vi "KM_appendline.vi"(4 "Time (s)":dbl, 6 "name or relative path":string, 7 "read/write control":T3, 8 "Field":dbl, 9 "temperature":dbl, 10 "pm lorentzian":T1={"Amplitude"=nan, "omega(0)"=47559.741592685685, "Gamma"=1.85203362605106e-05, "phase"=nan, "Q"=2567973978.6417074, "Norm  Ampl"=nan, "z (inf)"=nan+nani, "4corners"={"z (-pi/2)"=nan+nani, "z(inf)"=nan+nani, "z (pi/2)"=nan+nani, "z center"=nan+nani, "z(0)"=nan+nani, "radius"=nan}} {"z (inf)" format="%#9_9f"; "Q" format="%#9_9f"; "phase" format="%#9_9f"; "Gamma" format="%#9_9f"; "omega(0)" format="%#9_9f"}, 11 "Save frequency scan":path=path "C:/data/Ultrasound/birdcage/Hg1201/Test") -> ()   [LabVIEW 2016]
uses:
  KM_file -- read-write control.ctl
  lorentzian.ctl
  circle corners.ctl
  file -- read-write control.ctl
  <vilib>/Utility/libraryn.llb/Check if File or Folder Exists.vi
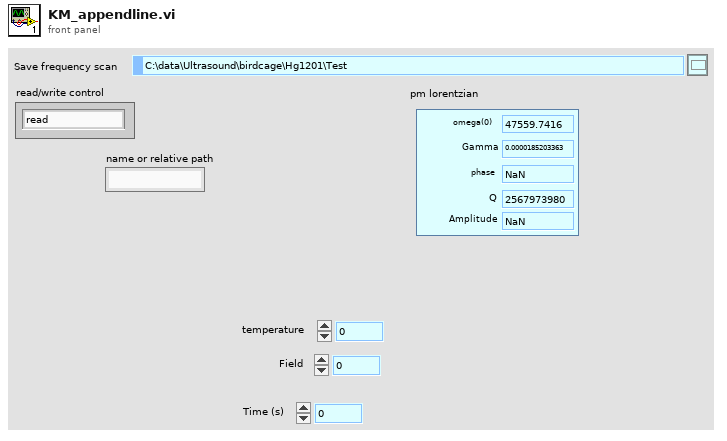
[diagram p1: front panel]
types:
  T1 = typedef "lorentzian.ctl" = cluster{"Amplitude":dbl, "omega(0)":dbl, "Gamma":dbl, "phase":dbl, "Q":dbl, "Norm  Ampl":dbl, "z (inf)":cdb, "4corners":T2}
  T2 = typedef "circle corners.ctl" = cluster{"z (-pi/2)":cdb, "z(inf)":cdb, "z (pi/2)":cdb, "z center":cdb, "z(0)":cdb, "radius":dbl}
  T3 = typedef "KM_file -- read-write control.ctl" = enum16{"read", "write all", "append one line"}
  T4 = typedef "file -- read-write control.ctl" = enum16{"read", "write all", "append one line"}
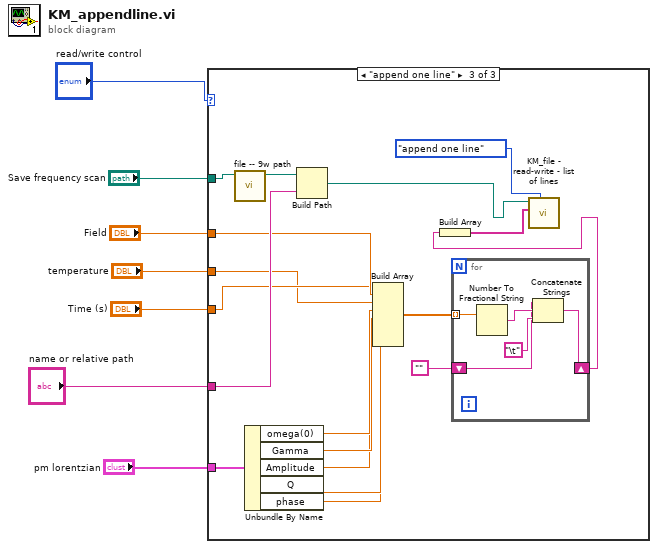
[diagram p0: block diagram]
diagram:
  n1 = case shown="\"append one line\"" "read/write control" {
    tunnel: "Save frequency scan" -> [_ _ w25]
    tunnel: "name or relative path" -> [_ _ w23]
    tunnel: "pm lorentzian" -> [_ _ w22]
    tunnel: "Field" -> [_ _ w21]
    tunnel: "Time (s)" -> [_ _ w20]
    tunnel: "temperature" -> [_ _ w19]
    frame "read", Default {
    }
    frame "write all" {
    }
    frame "append one line" {
      n2 = call "file -- 9w path.vi"("sweep folder"=w25) -> ("9w path"=w24:path)  [unwired: 10 in]
      n3 = Unbundle By Name(w22) -> ("omega(0)"=w18:dbl, "Gamma"=w17:dbl, "Amplitude"=w16:dbl, "Q"=w15:dbl, "phase"=w14:dbl)
      n4 = Build Path(base path=w24, name or relative path=w23) -> (appended path=w9:path)
      n5 = Build Array(w20, w21, w19, w18, w17, w16, w15, w14) -> (w13:dbl[])
      n6 = for {
        tunnel: w13 -> [w30] mode=indexing
        shift-right: [w26] -> w11
        shift-left: "" -> [w27]
        n7 = Number To Fractional String(number=w30) -> (F-format string=w29:string)  [unwired: 3 in]
        n8 = Concatenate Strings(w27, w29, "\t" ("string")) -> (w26:string)
      }
      n9 = Build Array(w11) -> (w8:string[])
      n10 = call "KM_file - read-write - list of lines.vi"("read/write control"=file_--_read-write_control."append one line", "list of lines IN"=w8, "file path"=w9) -> ()  [unwired: 7 in, 2 out]
    }
  }
